vi "Read Circular Buffer.vi"(8 "error in (no error)":errorcluster, 11 "Data Plugin in":refnum<class "Data Plugin.lvclass">) -> (0 "error out":errorcluster, 2 "Circular Buffer":dbl[](array[numeric]), 3 "Data Plugin out":refnum<class "Data Plugin.lvclass">)   [LabVIEW 2017, in "Data Engine.lvlib" / "Data Plugin.lvclass"]
uses:
  Data Plugin.lvclass
  Data Plugin.lvclass/Data Plugin.ctl
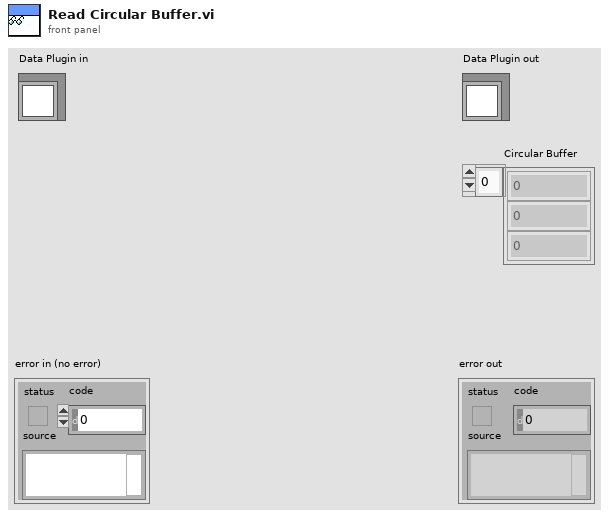
[diagram p1: front panel]
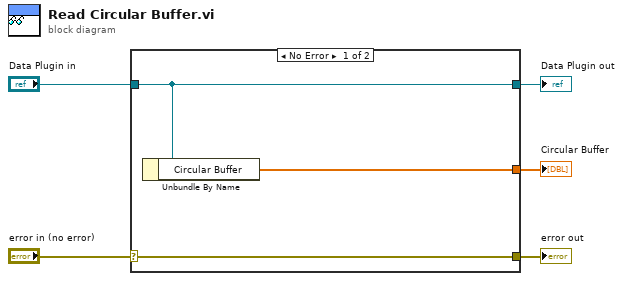
[diagram p0: block diagram]
diagram:
  n1 = case shown="No Error" "error in (no error)" {
    selector: "error in (no error)" -> [w8 w9]
    tunnel: [w8 w9] -> w4
    tunnel: [w7 w10] -> w2
    tunnel: "Data Plugin in" -> [w7 w10]
    tunnel: [w6 _] -> w1
    frame No Error {
      n2 = Unbundle By Name(w7) -> ("Circular Buffer"=w6:dbl[])
    }
    frame Error {
    }
  }
  "error out" <- w4
  "Data Plugin out" <- w2
  "Circular Buffer" <- w1
